vi "Create.vi"(0 "Serialized.EndStyle":T1, 5 "Serialized.FillColor":u32, 7 "Serialized.LineColor":u32) -> (4 "output cluster":refnum<class "FSM.EdgeEnd.lvclass">)   [LabVIEW 2020, in "FSM.EdgeEnd.lvclass"]
uses:
  FSM.EdgeEnd.lvclass
  EndStyle.ctl
  FSM.EdgeEnd.lvclass/FSM.EdgeEnd.ctl
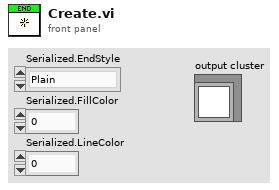
[diagram p1: front panel]
types:
  T1 = typedef "FSM.EdgeEnd.lvclass/EndStyle.ctl" = enum16{"Plain", "Arrow", "Box", "Circle", "Diamond"}
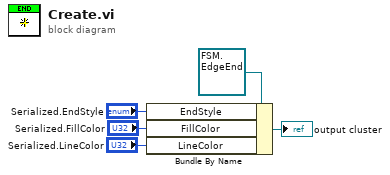
[diagram p0: block diagram]
diagram:
  n1 = Bundle By Name(cluster=refnum<class "FSM.EdgeEnd.lvclass"> refnum ("FSM.EdgeEnd"), "EndStyle"="Serialized.EndStyle", "FillColor"="Serialized.FillColor", "LineColor"="Serialized.LineColor") -> (→"output cluster":refnum<class "FSM.EdgeEnd.lvclass">)
